vi "disable_by_name.vi"(8 "error in (no error)":errorcluster caption="错误输入（无错误）", 10 "name":string, 11 "MotorSystem 输入":refnum<class "MotorSystem.lvclass">) -> (0 "error out":errorcluster caption="错误输出", 3 "MotorSystem 输出":refnum<class "MotorSystem.lvclass">)   [LabVIEW 2016, in "MotionControl.lvlib" / "MotorSystem.lvclass"]
uses:
  <userlib>/MotionControl/MotorSystem/MotorSystem.lvclass
  <userlib>/MotionControl/MotorSystem/MotorSystem.lvclass/MotorSystem.ctl
  <userlib>/MotionControl/OneMotion/OneMotion.lvclass
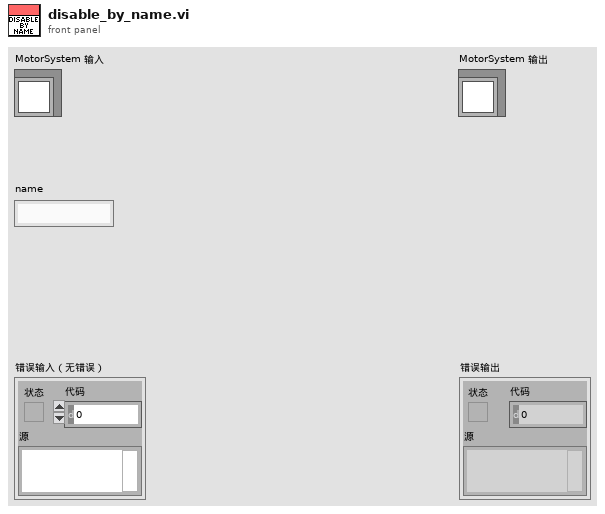
[diagram p1: front panel]
types:
  T1 = typedef "MotionControl.lvlib/MotorSystem.lvclass/MotionCluster.ctl" = cluster{"OneMotion.lvclass":refnum<class "OneMotion.lvclass">, "connected?":bool, "default enabled?":bool, "enabled?":bool}
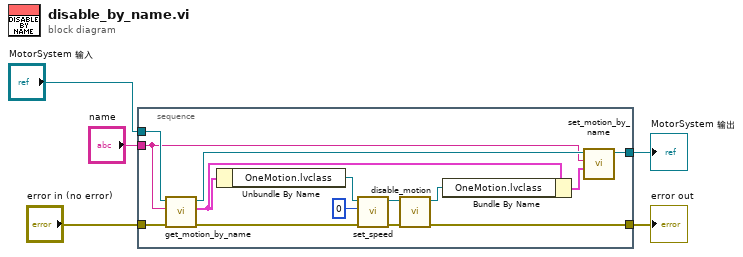
[diagram p0: block diagram]
diagram:
  n1 = stacked-sequence {
    tunnel: [w18] -> w5
    tunnel: [w15] -> w3
    tunnel: "MotorSystem 输入" -> [w17]
    tunnel: "error in (no error)" -> [w19]
    tunnel: "name" -> [w14]
    frame #0 {
      n2 = call <userlib>:"get_motion_by_name.vi"("error in (no error)"=w19, "name"=w14, "MotorSystem in"=w17) -> ("error out"=w7:errorcluster, "motion cluster"=w13:T1, "MotorSystem out"=w16:refnum<class "MotorSystem.lvclass">)  [unwired: 6 in]
      n3 = Unbundle By Name(w13) -> ("OneMotion.lvclass"=w10:refnum<class "OneMotion.lvclass">)
      n4 = call-dynamic "set_speed.vi"("error in (no error)"=w7, "speed"=0, "OneMotion 输入"=w10) -> ("error out"=w6:errorcluster, "OneMotion 输出"=w8:refnum<class "OneMotion.lvclass">)  [unwired: 7 in]
      n5 = call <userlib>:"disable_motion.vi"("error in (no error)"=w6, "OneMotion 输入"=w8) -> ("error out"=w18:errorcluster, "OneMotion 输出"=w12:refnum<class "OneMotion.lvclass">)  [unwired: 8 in]
      n6 = Bundle By Name(cluster=w13, "OneMotion.lvclass"=w12) -> (w11:T1)
      n7 = call <userlib>:"set_motion_by_name.vi"("簇"=w11, "name"=w14, "MotorSystem输入"=w16) -> ("MotorSystem输出"=w15:refnum<class "MotorSystem.lvclass">)  [unwired: 7 in, 1 out]
    }
  }
  "error out" <- w5
  "MotorSystem 输出" <- w3
